vi "Set URI String.vi"(8 "error in (no error)":errorcluster, 10 "URI String":string, 11 "Endpoint in":refnum<class "Endpoint.lvclass">) -> (0 "error out":errorcluster, 3 "Endpoint out":refnum<class "Endpoint.lvclass">)   [LabVIEW 2020, in "Stream.lvlib" / "Endpoint.lvclass"]
uses:
  Endpoint.lvclass
  Endpoint.lvclass/Endpoint.ctl
  URI/URI.lvclass
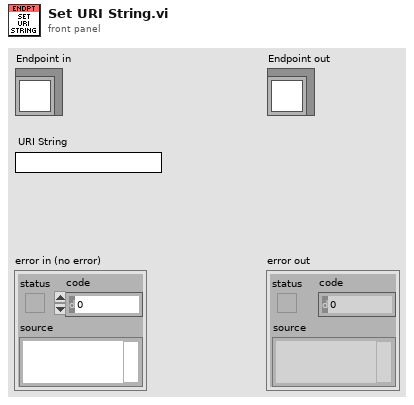
[diagram p1: front panel]
types:
  T1 = typedef "Stream.lvlib/Endpoint.lvclass/Ref Data.ctl" = cluster{"URI":refnum<class "URI.lvclass">, "State Callbacks":T2[]}
  T2 = typedef "Stream.lvlib/Endpoint.lvclass/State Callback.ctl" = cluster{"Owner":refnum<class>, "VI":refnum<vi>}
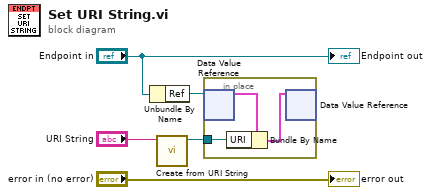
[diagram p0: block diagram]
diagram:
  n1 = Unbundle By Name("Endpoint in") -> ("Ref"=w3:refnum<data-value>)
  n2 = call "Create from URI String.vi"("URI String"="URI String") -> ("URI out"=w1:refnum<class "URI.lvclass">)  [unwired: 9 in, 1 out]
  n3 = in-place {
    in-place-border: w1 -> [w6]
    n4 = in-place-dvr #1(w3) -> (w8:T1)  [unwired: 1 out]
    n5 = Bundle By Name(cluster=w8, "URI"=w6) -> (w7:T1)
    n6 = in-place-dvr #1(w7) -> ()  [unwired: 2 out]
  }
  "error out" <- "error in (no error)"
  "Endpoint out" <- "Endpoint in"
